vi "Batch Editor Dialog.vi"(5 "VI Refnum":refnum<vi>, 6 "Listbox":refnum<vi>, 7 "Reference":variant, 8 "Error in":errorcluster caption="Error in (no error)", 9 "Option":variant, 10 "Root":path, 11 "Entries":string[](array[string])) -> (0 "Error out":errorcluster)   [LabVIEW 2017, in "batchEditorDialog.lvlib"]
uses:
  batchEditorDialog.lvlib
  _Shared/CSM Shared.lvlib
panel:
  out "Listbox":i32(listbox)
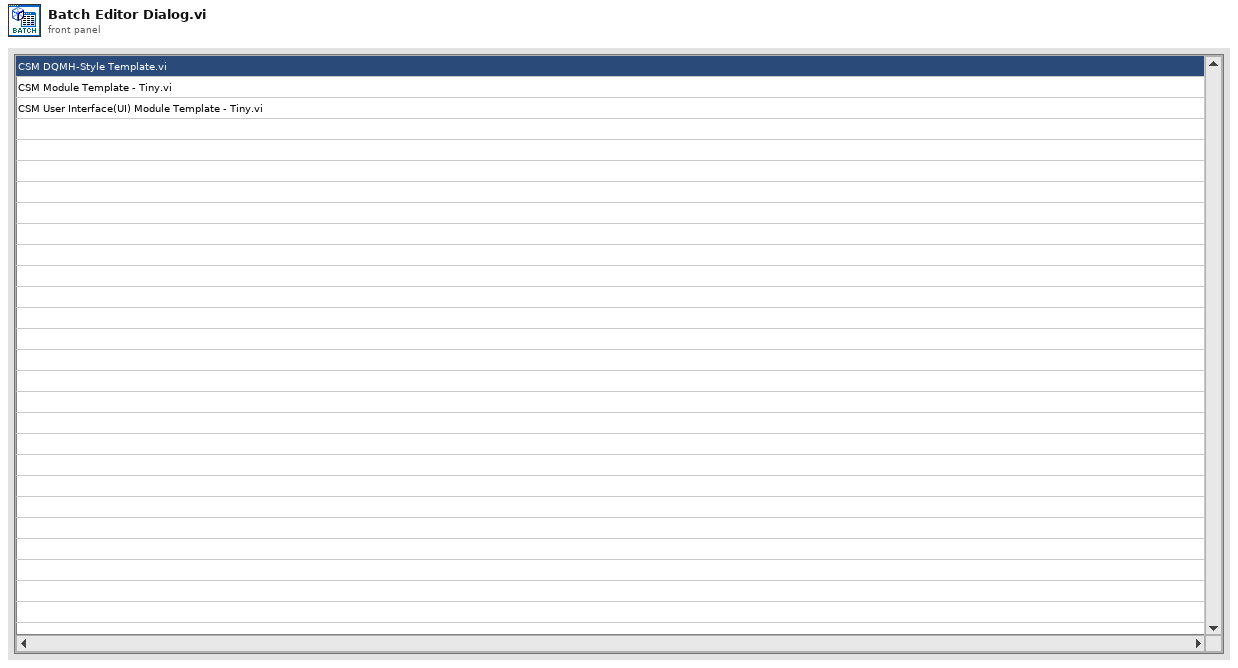
[diagram p1: front panel]
types:
  T1 = enum32{"Invalid", "Standard", "Closed", "Hidden", "Minimized", "Maximized"}
  T2 = enum32{"invalid app kind", "Development System", "Run Time System", "Student Edition", "Embedded LabVIEW", "Evaluation", "Custom"}
  T3 = cluster{"Core":cluster{"Current VI Reference":refnum<vi>, "Close Panel on Exit?":bool}, "Entries":string[], "Success":bool, "Listbox":refnum<vi>}
  T4 = cluster{"Current VI Reference":refnum<vi>, "Close Panel on Exit?":bool}
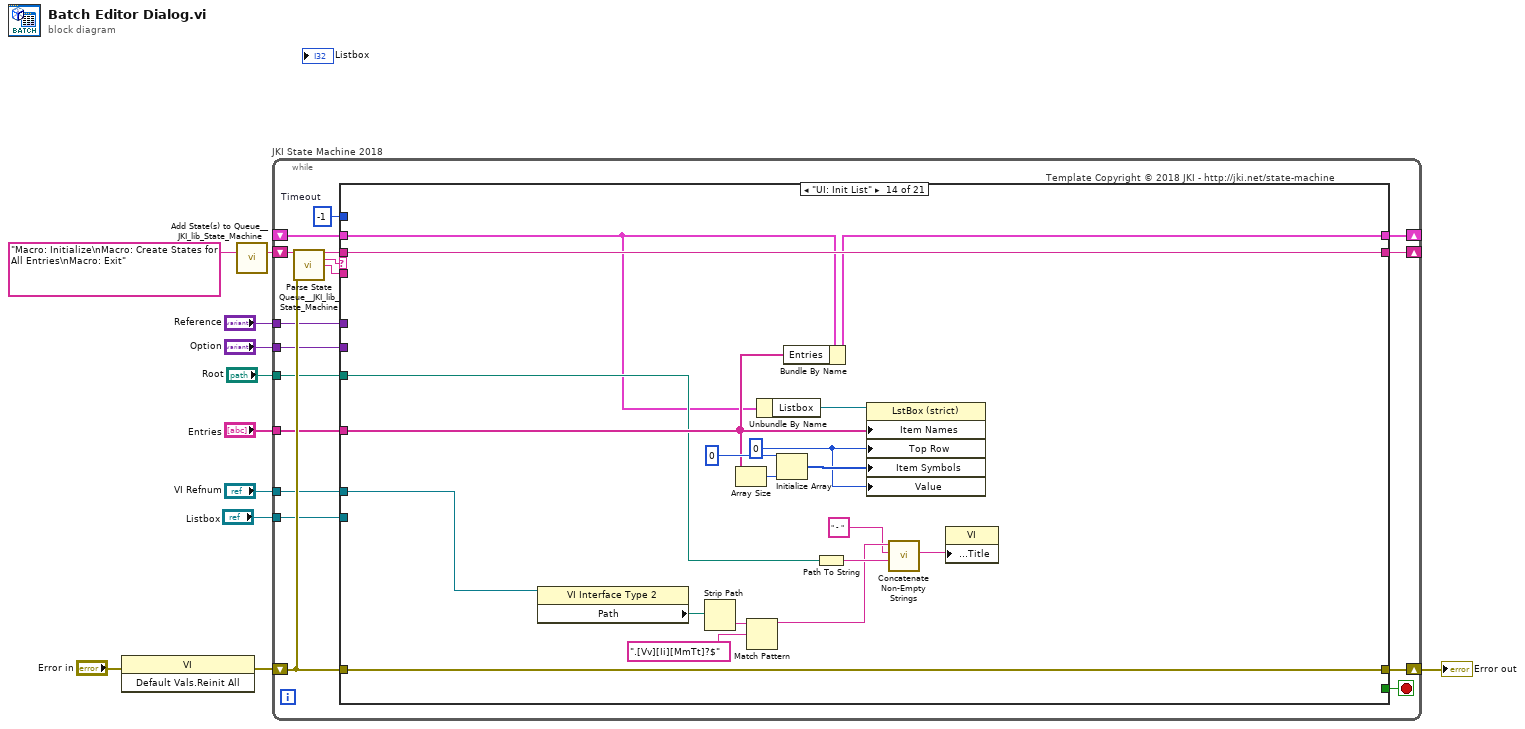
[diagram p0: block diagram]
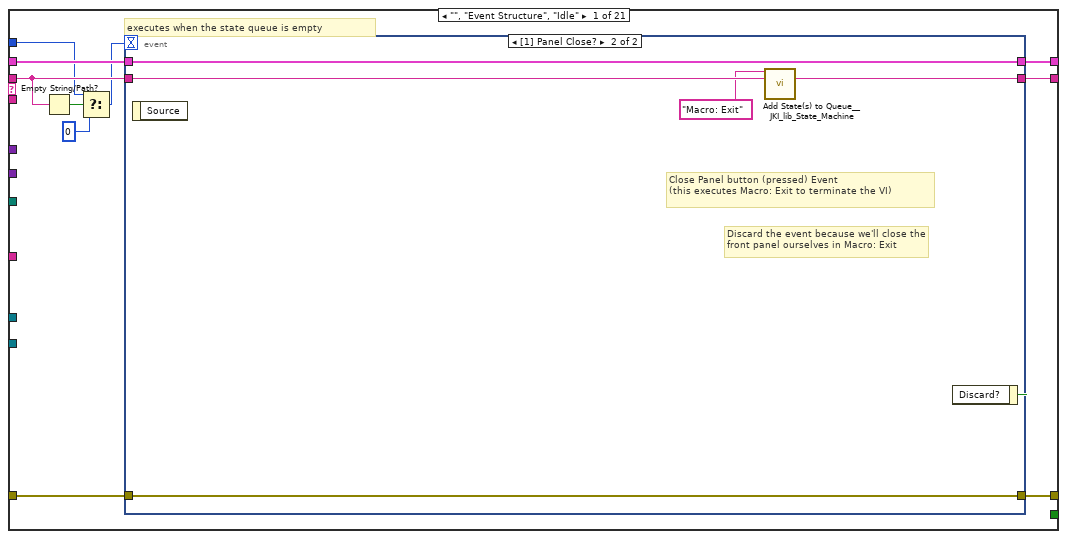
[diagram p2: hidden frame]
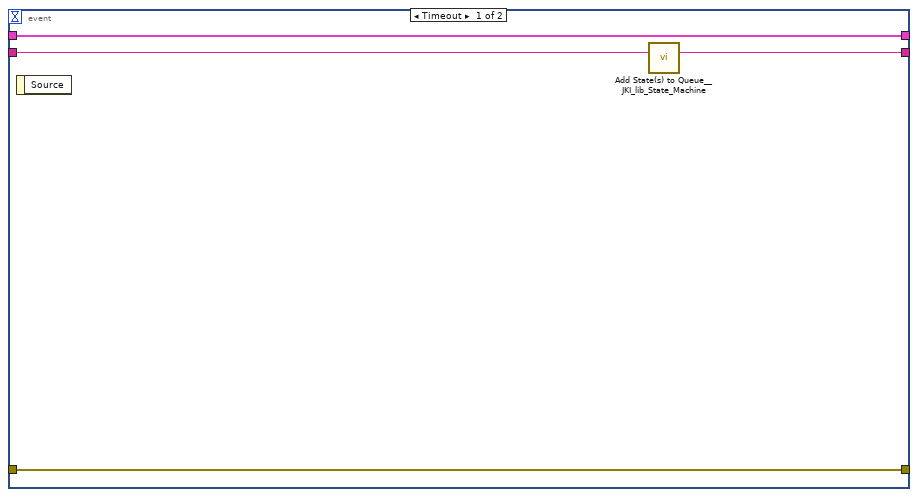
[diagram p3: hidden frame]
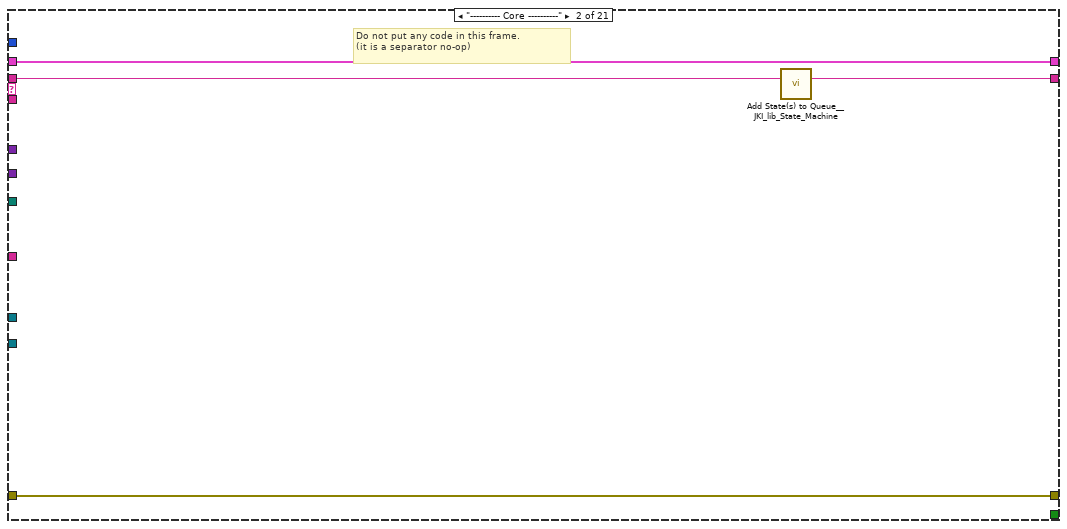
[diagram p4: hidden frame]
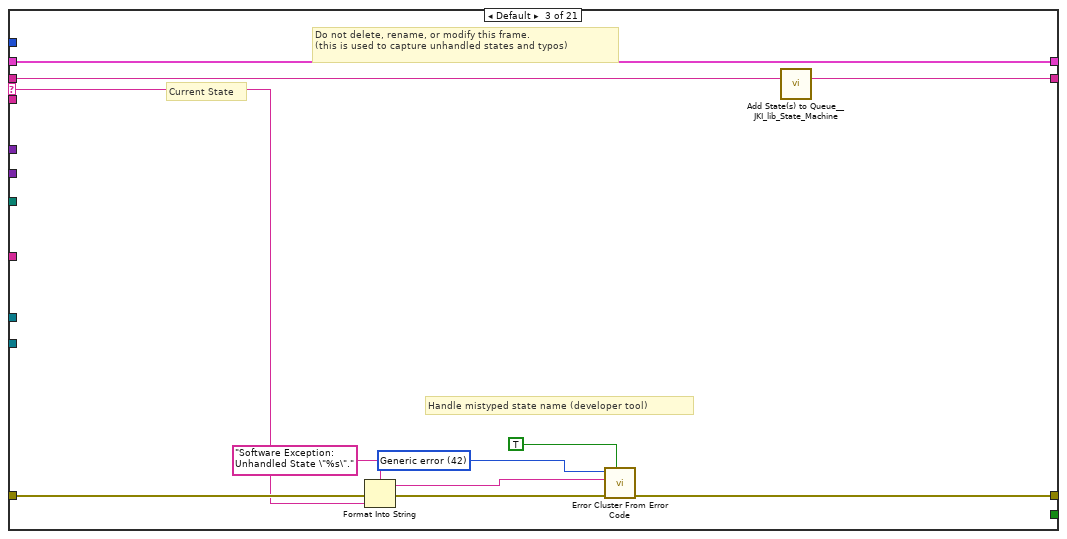
[diagram p5: hidden frame]
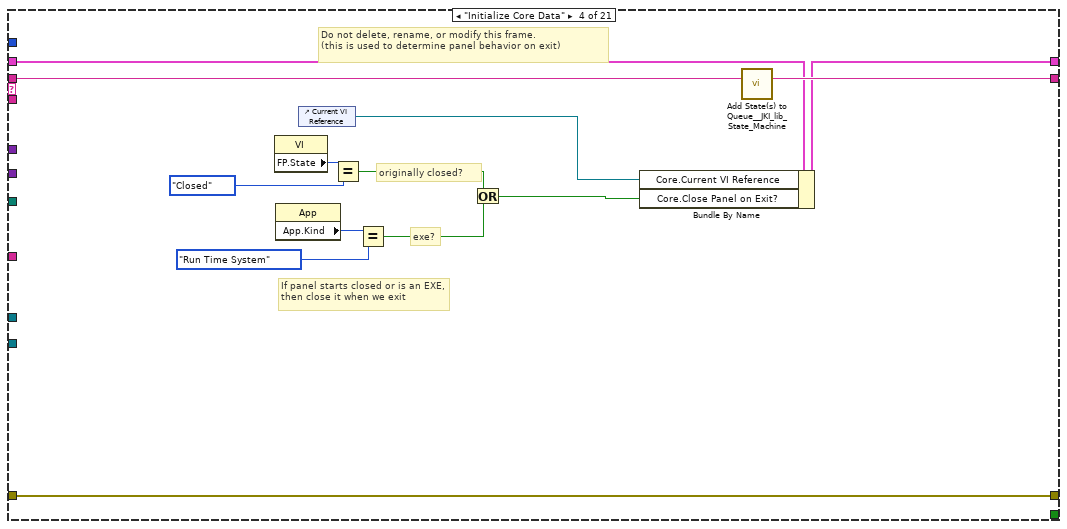
[diagram p6: hidden frame]
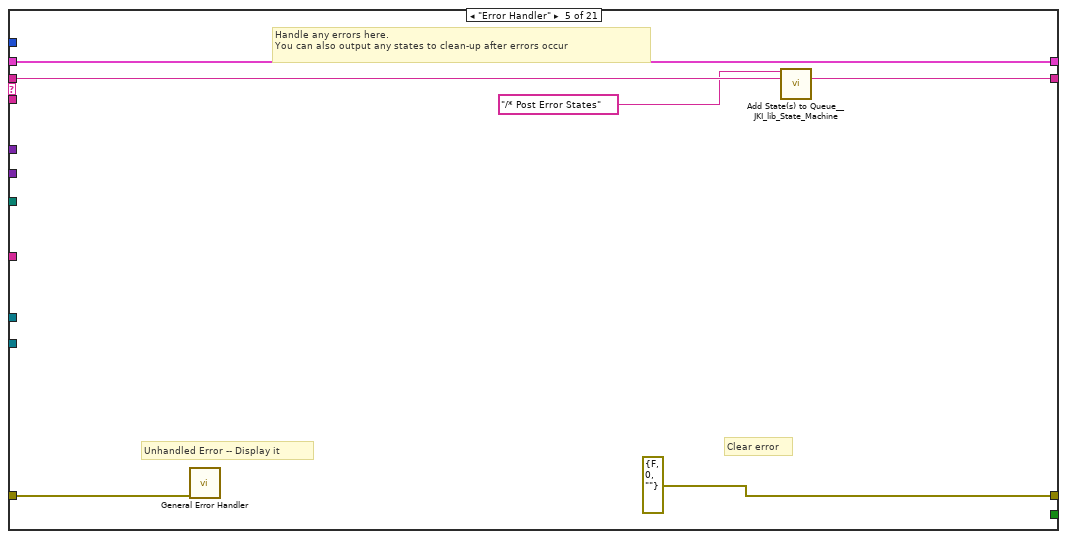
[diagram p7: hidden frame]
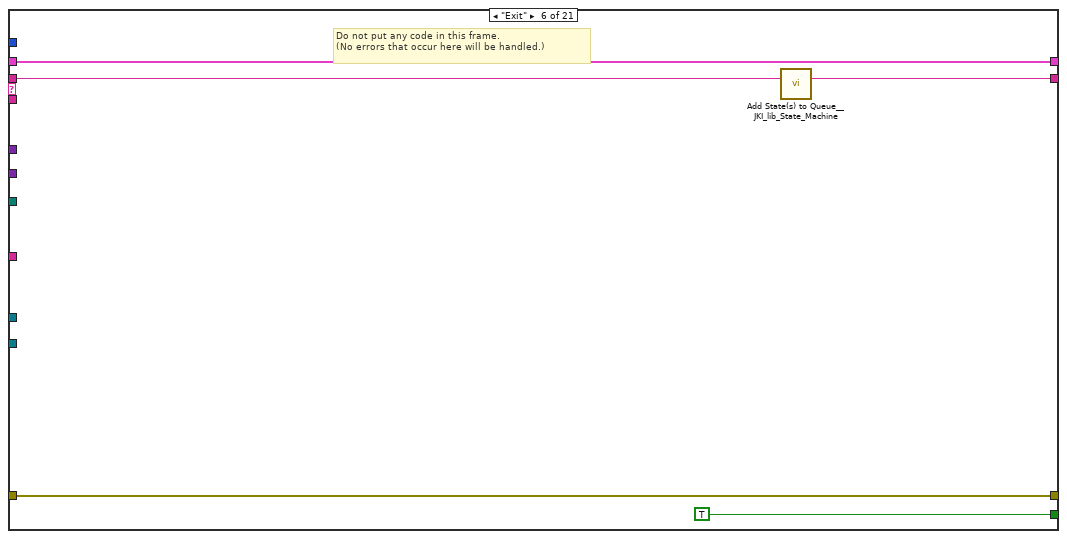
[diagram p8: hidden frame]
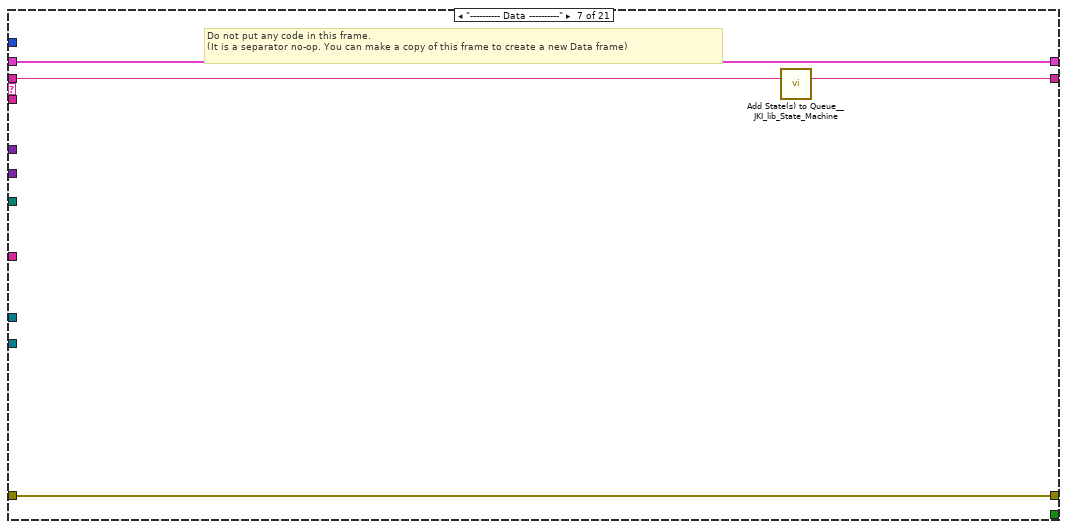
[diagram p9: hidden frame]
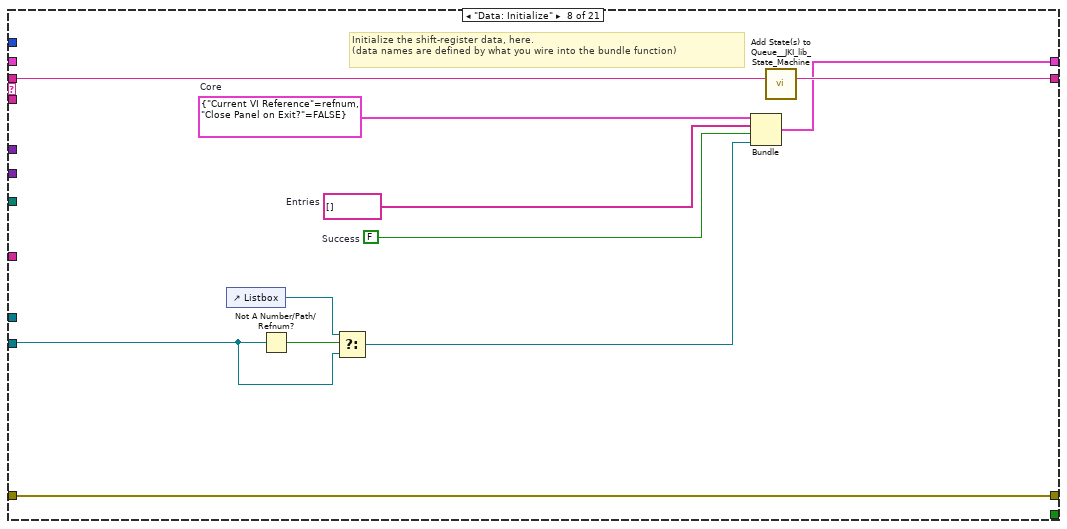
[diagram p10: hidden frame]
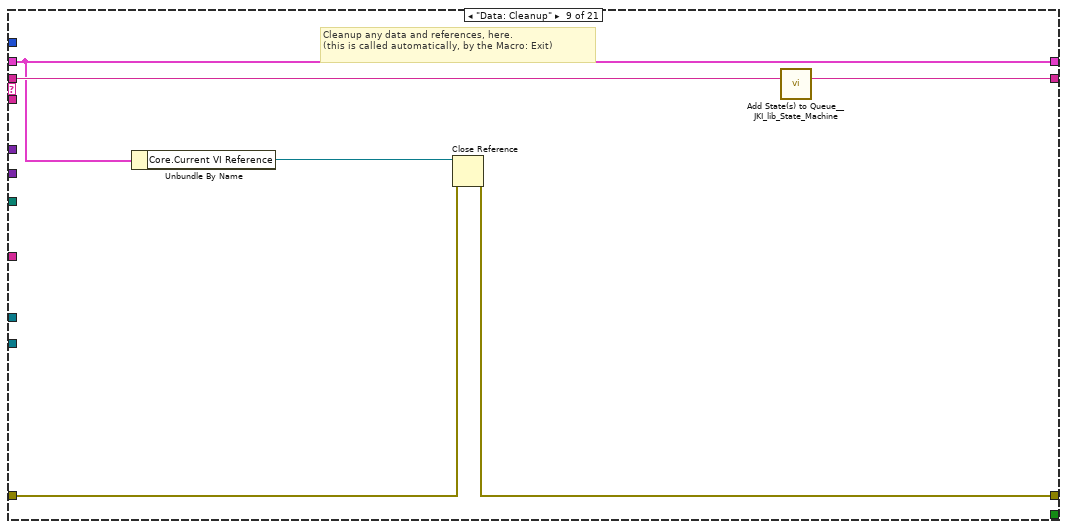
[diagram p11: hidden frame]
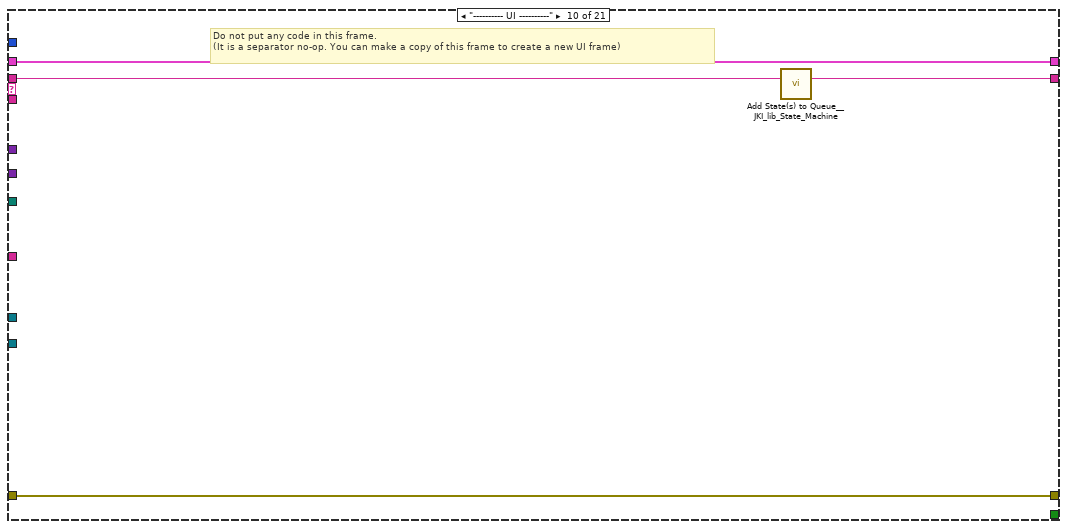
[diagram p12: hidden frame]
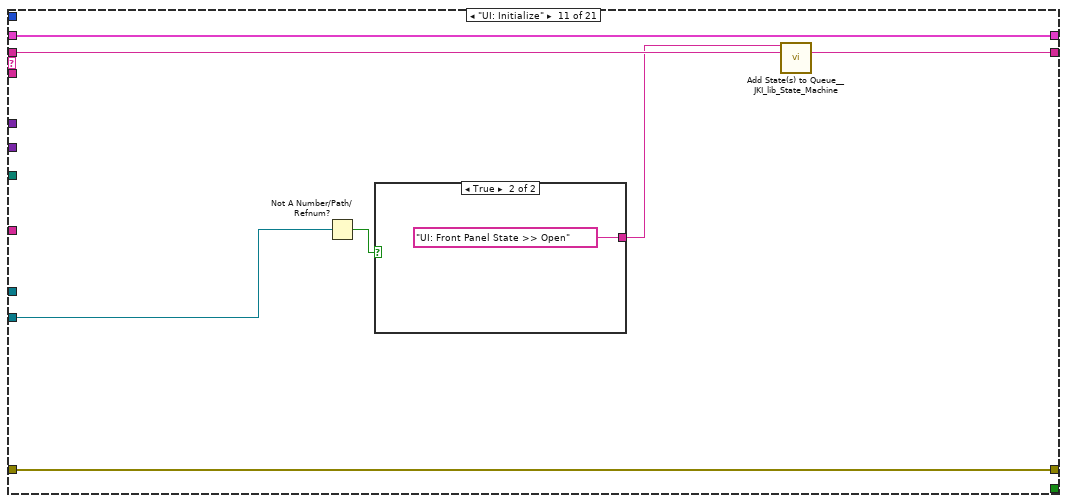
[diagram p13: hidden frame]
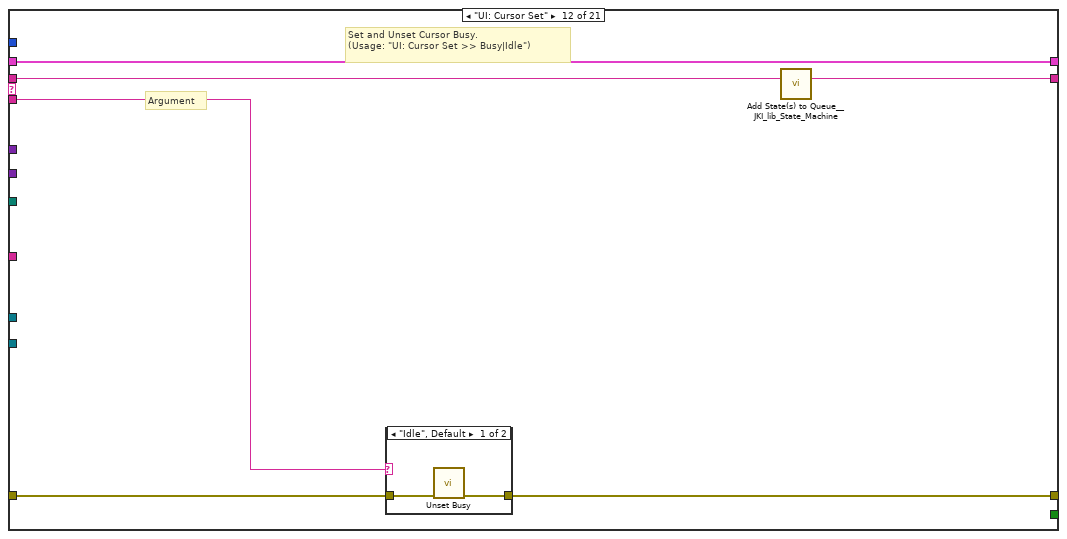
[diagram p15: hidden frame]
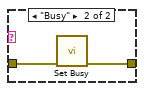
[diagram p16: hidden frame]
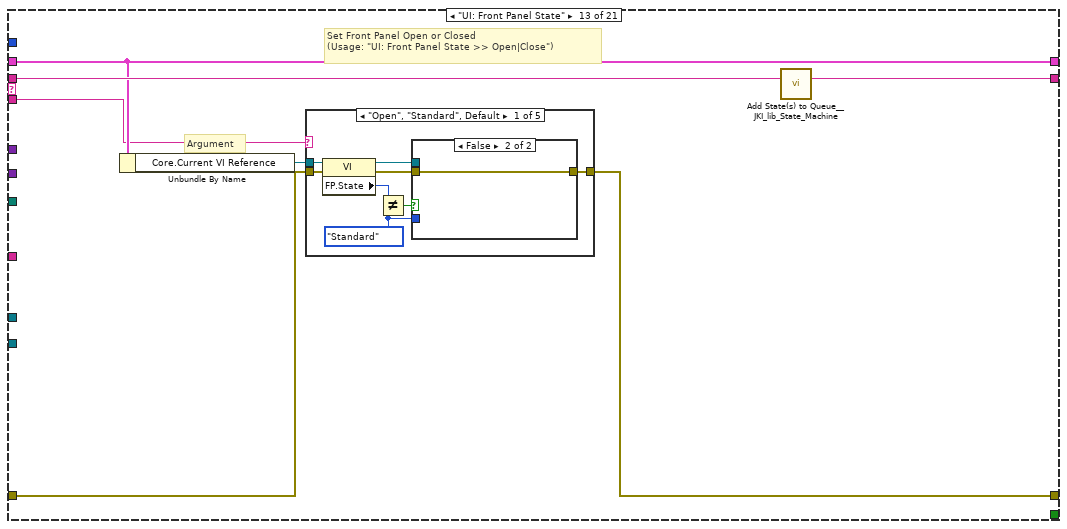
[diagram p17: hidden frame]
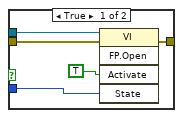
[diagram p18: hidden frame]
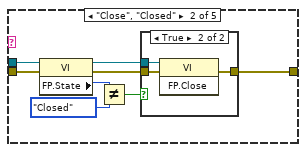
[diagram p19: hidden frame]
diagram:
  n1 = invoke class="VI" method="Default Vals.Reinit All"(error in="Error in") -> (error out=w9:errorcluster)  [unwired: 2 in, 2 out]
  n2 = call <vilib>:"Add State(s) to Queue__JKI_lib_State_Machine.vi"("State(s) in (\"\")"="Macro: Initialize\nMacro: Create States for All Entries\nMacro: Exit") -> ("States Out"=w11:string)  [unwired: 14 in]
  n3 = while "JKI State Machine 2018" {
    shift-right: [w21] -> _
    shift-left: _ -> [w20]
    shift-right: [w24] -> w7
    shift-left: w9 -> [w18]
    shift-right: [w23] -> _
    shift-left: w11 -> [w25]
    tunnel: "Reference" -> [w17]
    tunnel: "Option" -> [w16]
    tunnel: "Entries" -> [w15]
    tunnel: "VI Refnum" -> [w14]
    tunnel: "Root" -> [w13]
    tunnel: "Listbox" -> [w12]
    stop <- w22 stop-if-true
    w19 = -1  # Timeout
    # "Template Copyright © 2018 JKI - http://jki.net/state-machine"
    n4 = call <vilib>:"Parse State Queue__JKI_lib_State_Machine.vi"("State Queue"=w25, "Error In (no error)"=w18) -> ("Remaining States"=w27:string, "Current State"=w28:string, "Arguments"=w26:string)  [unwired: 11 in]
    n5 = case shown="\"UI: Init List\"" w28 {
      selector: w28 -> [_ _ w53 _ _ _ _ _ _ _ _ _ _ _ _ _ _ _ _ _ _]
      tunnel: w27 -> [w33 w52 w57 w76 w82 w87 w91 w102 w108 w112 w119 w126 w137 w220 w225 w247 w252 w262 w266 w274 w292]
      tunnel: w26 -> [_ _ _ _ _ _ _ _ _ _ _ w121 w131 _ _ _ _ _ _ _ w286]
      tunnel: w20 -> [w37 w49 w55 w69 w79 w85 w88 _ w103 w109 w116 w124 w133 w212 w223 w244 w249 w259 w263 w270 w290]
      tunnel: [w36 w50 w59 w73 errorcluster {"status"=FALSE, "code"=0, "source"=""} ("error out") w84 w89 w99 w104 w110 w117 w122 w134 w221 w243 w245 w250 w260 w264 w272 _] -> w24
      tunnel: w18 -> [w35 w50 w58 w73 w78 w84 w89 w99 w105 w110 w117 w123 w135 w221 w243 w245 w250 w260 w264 w272 _]
      tunnel: [w38 w51 w56 w75 w81 w86 w90 w101 w107 w111 w118 w125 w136 w220 w226 w246 w251 w261 w265 w273 w293] -> w23
      tunnel: [_ _ _ _ _ TRUE _ _ _ _ _ _ _ _ _ _ _ _ _ _ _] -> w22
      tunnel: [w34 w49 w55 w74 w79 w85 w88 w100 w103 w109 w116 w124 w133 w215 w232 w244 w249 w259 w263 w270 w295] -> w21
      tunnel: w19 -> [w32 _ _ _ _ _ _ _ _ _ _ _ _ _ _ _ _ _ _ _ _]
      tunnel: w17 -> [_ _ _ _ _ _ _ _ _ _ _ _ _ _ _ _ _ _ _ _ w285]
      tunnel: w16 -> [_ _ _ _ _ _ _ _ _ _ _ _ _ _ _ _ _ _ _ _ w284]
      tunnel: w15 -> [_ _ _ _ _ _ _ _ _ _ _ _ _ w214 _ _ _ _ _ _ _]
      tunnel: w14 -> [_ _ _ _ _ _ _ _ _ _ _ _ _ w210 _ _ _ _ _ _ w283]
      tunnel: w13 -> [_ _ _ _ _ _ _ _ _ _ _ _ _ w213 _ _ _ _ _ _ w281]
      tunnel: w12 -> [_ _ _ _ _ _ _ w93 _ _ w114 _ _ _ _ _ _ _ _ _ _]
      frame "", "Event Structure", "Idle" {
        # "executes when the state queue is empty"
        n6 = Empty String/Path?(string/path=w33) -> (empty?=w30:bool)
        n7 = Select(t=w32, s=w30, f=0) -> (s? t:f=w31:i32)
        n8 = event shown="[1] Panel Close?" {
          selector: _ -> [_ _]
          dyn-events: _ -> [_ _]
          timeout: w31 -> [_ _]
          tunnel: w33 -> [w42 w48]
          tunnel: [w41 w47] -> w38
          tunnel: w37 -> [w39 w45]
          tunnel: [w40 w46] -> w36
          tunnel: w35 -> [w40 w46]
          tunnel: [w39 w45] -> w34
          event Timeout {
            n9 = event-data() -> ()  [unwired: 1 in, 1 out]
            n10 = call <vilib>:"Add State(s) to Queue__JKI_lib_State_Machine.vi"("State(s) in (\"\")"=w42) -> ("States Out"=w41:string)  [unwired: 14 in]
          }
          event Panel Close? {
            # "Discard the event because we'll close the front panel ourselves in Macro: Exit"
            # "Close Panel button (pressed) Event\n(this executes Macro: Exit to terminate the VI)"
            n11 = event-data() -> ()  [unwired: 1 in, 1 out]
            n12 = call <vilib>:"Add State(s) to Queue__JKI_lib_State_Machine.vi"("State(s) in Front (\"\")"="Macro: Exit", "State(s) in (\"\")"=w48) -> ("States Out"=w47:string)  [unwired: 13 in]
            n13 = event-data("Discard?"=TRUE) -> ()  [unwired: 1 in, 1 out]
          }
        }
      }
      frame "---------- Core ----------" {
        # "Do not put any code in this frame.\n(it is a separator no-op)"
        n14 = call <vilib>:"Add State(s) to Queue__JKI_lib_State_Machine.vi"("State(s) in (\"\")"=w52) -> ("States Out"=w51:string)  [unwired: 14 in]
      }
      frame Default {
        w62 = 42 items=["No error", "Argument error", "Memory is full", "Out of zone", "End of file", "File already open", "Generic file I/O error", "File not found", "File permission error", "Disk is full", "Duplicate path", "Too many files open", "System feature not enabled", "Resource file not found", "Cannot add resource", "Resource not found", "Image not found", "Image memory error", "Pen does not exist", "Config type invalid", "Config token not found", "Config parse error", "Config memory error", "Bad external code format", "Bad external code offset", "External code not present", "Null window", "Destroy window error", "Null menu", "Print aborted", "Bad print record", "Print driver error", "Windows error during printing", "Memory error during printing", "Print dialog error", "Generic print error", "Invalid device refnum", "Device not found", "Device parameter error", "Device unit error", "Cannot open device", "Device call aborted", "Generic error", "Cancelled by user", "Object ID too low", "Object ID too high", "Object not in heap", "Unknown heap", "Unknown object (invalid DefProc)", "Unknown object (DefProc not in table)", "Message out of range", "Invalid (null) method", "Unknown message", "Manager call not supported", "Bad address", "Network operation in progress", "Network operation timed out", "Connection is busy", "Network attribute not supported", "Network error", "Address in use", "System out of memory", "Connection aborted", "Connection refused", "Not connected", "Already connected", "Connection closed", "Initialization error (interapplication manager)", "Bad occurrence", "Wait on unbound occurrence handler", "Occurrence queue overflow", "Datalog type conflict", "Unused", "Unrecognized type (interapplication manager)", "Memory corrupt", "Failed to make temporary DLL", "Old CIN version", "Drag socket not found", "Failed to load drop-object", "Failed to register OLE object", "Failed to release OLE object", "Format specifier type mismatch", "Unknown format specifier", "Too few format specifiers", "Too many format specifiers", "Scan failed", "Newer CIN version", "Error converting to variant", "Runtime menu error", "Password tampered", "Variant attribute not found", "Incompatible variant data type", "Event data is not available", "Event Store is not present", "Occurrence is not found", "Event Queue is not created", "Event info is not available", "Refnum passed is NULL", "Error retrieving Class GUID", "Error retrieving CoClass GUID", "Error retrieving TypeLib GUID.", "Bad built application magic bytes.", "Specific driver is different from the specific driver associated with the Logical Name.", "There is no session opened to the class driver.", "Max Error", "MAX - Error with config objects", "MAX - Error loading configuration", "MAX - Group not supported"]
        # "Current State"
        # "Do not delete, rename, or modify this frame.\n(this is used to capture unhandled states and typos)"
        # "Handle mistyped state name (developer tool)"
        n15 = Format Into String(format string="Software Exception: Unhandled State \"%s\"." ("message"), error in=w58, w53) -> (resulting string=w61:string, error out=w60:errorcluster)  [unwired: 1 in]
        n16 = call <vilib>:"Error Cluster From Error Code.vi"("show call chain? (False)"=TRUE, "error in (no error)"=w60, "error message (\"\")"=w61, "error code (0)"=w62) -> ("error out"=w59:errorcluster)  [unwired: 5 in]
        n17 = call <vilib>:"Add State(s) to Queue__JKI_lib_State_Machine.vi"("State(s) in (\"\")"=w57) -> ("States Out"=w56:string)  [unwired: 14 in]
      }
      frame "Initialize Core Data" {
        # "Do not delete, rename, or modify this frame.\n(this is used to determine panel behavior on exit)"
        # "originally closed?"
        # "exe?"
        # "If panel starts closed or is an EXE, then close it when we exit"
        n18 = property class="VI"() -> ("FP.State"=w66:T1)  [unwired: 2 in, 2 out]
        n19 = property class="App"() -> ("App.Kind"=w72:T2)  [unwired: 2 in, 2 out]
        n20 = control-ref of="Current VI Reference"() -> (w67:refnum<vi>)
        n21 = Equal?(x=w66, y=T1."Closed" ("Front Panel Window:State")) -> (x = y?=w64:bool)
        n22 = Equal?(x=w72, y=T2."Run Time System" ("Application:Kind")) -> (x = y?=w70:bool)
        n23 = Or(x=w64, y=w70) -> (x .or. y?=w68:bool)
        n24 = Bundle By Name(cluster=w69, "Core.Current VI Reference"=w67, "Core.Close Panel on Exit?"=w68) -> (w74:T3)
        n25 = call <vilib>:"Add State(s) to Queue__JKI_lib_State_Machine.vi"("State(s) in (\"\")"=w76) -> ("States Out"=w75:string)  [unwired: 14 in]
      }
      frame "Error Handler" {
        # "Unhandled Error -- Display it"
        # "Handle any errors here.\nYou can also output any states to clean-up after errors occur"
        # "Clear error"
        n26 = call <vilib>:"General Error Handler.vi"("error in (no error)"=w78) -> ()  [unwired: 10 in, 5 out]
        n27 = call <vilib>:"Add State(s) to Queue__JKI_lib_State_Machine.vi"("State(s) in Front (\"\")"="/* Post Error States", "State(s) in (\"\")"=w82) -> ("States Out"=w81:string)  [unwired: 13 in]
      }
      frame "Exit" {
        # "Do not put any code in this frame.\n(No errors that occur here will be handled.)"
        n28 = call <vilib>:"Add State(s) to Queue__JKI_lib_State_Machine.vi"("State(s) in (\"\")"=w87) -> ("States Out"=w86:string)  [unwired: 14 in]
      }
      frame "---------- Data ----------" {
        # "Do not put any code in this frame.\n(It is a separator no-op. You can make a copy of this frame to create a new Data frame)"
        n29 = call <vilib>:"Add State(s) to Queue__JKI_lib_State_Machine.vi"("State(s) in (\"\")"=w91) -> ("States Out"=w90:string)  [unwired: 14 in]
      }
      frame "Data: Initialize" {
        w96 = FALSE  # Success
        w97 = string[] []  # Entries
        w98 = T4 {"Current VI Reference"=refnum, "Close Panel on Exit?"=FALSE}  # Core
        # "Initialize the shift-register data, here.\n(data names are defined by what you wire into the bundle function)"
        n30 = control-ref of="Listbox"() -> (w94:refnum<vi>)
        n31 = Not A Number/Path/Refnum?(number/path/refnum=w93) -> (NaN/Path/Refnum?=w95:bool)
        n32 = Select(t=w94, s=w95, f=w93) -> (s? t:f=w92:refnum<vi>)
        n33 = Bundle("Core"=w98, "Entries"=w97, "Success"=w96, "Listbox"=w92) -> (w100:T3)  [unwired: 1 in]
        n34 = call <vilib>:"Add State(s) to Queue__JKI_lib_State_Machine.vi"("State(s) in (\"\")"=w102) -> ("States Out"=w101:string)  [unwired: 14 in]
      }
      frame "Data: Cleanup" {
        # "Cleanup any data and references, here.\n(this is called automatically, by the Macro: Exit)"
        n35 = Unbundle By Name(w103) -> ("Core.Current VI Reference"=w106:refnum<vi>)
        n36 = Close Reference(reference=w106, error in (no error)=w105) -> (error out=w104:errorcluster)
        n37 = call <vilib>:"Add State(s) to Queue__JKI_lib_State_Machine.vi"("State(s) in (\"\")"=w108) -> ("States Out"=w107:string)  [unwired: 14 in]
      }
      frame "---------- UI ----------" {
        # "Do not put any code in this frame.\n(It is a separator no-op. You can make a copy of this frame to create a new UI frame)"
        n38 = call <vilib>:"Add State(s) to Queue__JKI_lib_State_Machine.vi"("State(s) in (\"\")"=w112) -> ("States Out"=w111:string)  [unwired: 14 in]
      }
      frame "UI: Initialize" {
        n39 = Not A Number/Path/Refnum?(number/path/refnum=w114) -> (NaN/Path/Refnum?=w113:bool)
        n40 = case shown="True" w113 {
          tunnel: [_ "UI: Front Panel State >> Open" ("State(s) in Front (\"\")")] -> w115
          frame False {
          }
          frame True {
          }
        }
        n41 = call <vilib>:"Add State(s) to Queue__JKI_lib_State_Machine.vi"("State(s) in Front (\"\")"=w115, "State(s) in (\"\")"=w119) -> ("States Out"=w118:string)  [unwired: 13 in]
      }
      frame "UI: Cursor Set" {
        # "Argument"
        # "Set and Unset Cursor Busy.\n(Usage: \"UI: Cursor Set >> Busy|Idle\")"
        n42 = case shown="\"Idle\", Default" w121 {
          tunnel: w123 -> [w128 w130]
          tunnel: [w127 w129] -> w122
          frame "Idle", Default {
            n43 = call <vilib>:"Unset Busy.vi"("error in (no error)"=w128) -> ("error out"=w127:errorcluster)  [unwired: 10 in]
          }
          frame "Busy" {
            n44 = call <vilib>:"Set Busy.vi"("error in (no error)"=w130) -> ("error out"=w129:errorcluster)  [unwired: 9 in, 1 out]
          }
        }
        n45 = call <vilib>:"Add State(s) to Queue__JKI_lib_State_Machine.vi"("State(s) in (\"\")"=w126) -> ("States Out"=w125:string)  [unwired: 14 in]
      }
      frame "UI: Front Panel State" {
        # "Argument"
        # "Set Front Panel Open or Closed\n(Usage: \"UI: Front Panel State >> Open|Close\")"
        n46 = Unbundle By Name(w133) -> ("Core.Current VI Reference"=w132:refnum<vi>)
        n47 = case shown="\"Open\", \"Standard\", Default" w131 {
          tunnel: w135 -> [w143 w158 w169 w182 w195]
          tunnel: [w145 w159 w171 w184 w197] -> w134
          tunnel: w132 -> [w144 w156 w170 w183 w196]
          frame "Open", "Standard", Default {
            w138 = T1."Standard" ("State")
            n48 = property class="VI"(reference=w144, error in=w143) -> (reference out=w141:refnum<vi>, error out=w142:errorcluster, "FP.State"=w140:T1)
            n49 = Not Equal?(x=w140, y=w138) -> (x != y?=w139:bool)
            n50 = case shown="False" w139 {
              tunnel: [w149 w151] -> w145
              tunnel: w142 -> [w148 w151]
              tunnel: w141 -> [w147 _]
              tunnel: w138 -> [w146 _]
              frame True {
                n51 = invoke class="VI" method="FP.Open"(reference=w147, error in=w148, "Activate"=TRUE, "State"=w146) -> (error out=w149:errorcluster)  [unwired: 1 in, 4 out]
              }
              frame False {
              }
            }
          }
          frame "Close", "Closed" {
            n52 = property class="VI"(reference=w156, error in=w158) -> (reference out=w155:refnum<vi>, error out=w157:errorcluster, "FP.State"=w153:T1)
            n53 = Not Equal?(x=w153, y=T1."Closed" ("Front Panel Window:State")) -> (x != y?=w152:bool)
            n54 = case shown="True" w152 {
              tunnel: [w160 w163] -> w159
              tunnel: w157 -> [w160 w162]
              tunnel: w155 -> [_ w161]
              frame False {
              }
              frame True {
                n55 = invoke class="VI" method="FP.Close"(reference=w161, error in=w162) -> (error out=w163:errorcluster)  [unwired: 1 in, 2 out]
              }
            }
          }
          frame "Hidden", "Hide" {
            w164 = T1."Hidden" ("State")
            n56 = property class="VI"(reference=w170, error in=w169) -> (reference out=w167:refnum<vi>, error out=w168:errorcluster, "FP.State"=w166:T1)
            n57 = Not Equal?(x=w166, y=w164) -> (x != y?=w165:bool)
            n58 = case shown="True" w165 {
              tunnel: [w175 w176] -> w171
              tunnel: w168 -> [w174 w176]
              tunnel: w167 -> [w173 _]
              tunnel: w164 -> [w172 _]
              frame True {
                n59 = invoke class="VI" method="FP.Open"(reference=w173, error in=w174, "State"=w172) -> (error out=w175:errorcluster)  [unwired: 2 in, 4 out]
              }
              frame False {
              }
            }
          }
          frame "Minimize", "Minimized" {
            w177 = T1."Minimized" ("State")
            n60 = property class="VI"(reference=w183, error in=w182) -> (reference out=w180:refnum<vi>, error out=w181:errorcluster, "FP.State"=w179:T1)
            n61 = Not Equal?(x=w179, y=w177) -> (x != y?=w178:bool)
            n62 = case shown="True" w178 {
              tunnel: [w188 w189] -> w184
              tunnel: w181 -> [w187 w189]
              tunnel: w180 -> [w186 _]
              tunnel: w177 -> [w185 _]
              frame True {
                n63 = invoke class="VI" method="FP.Open"(reference=w186, error in=w187, "State"=w185) -> (error out=w188:errorcluster)  [unwired: 2 in, 4 out]
              }
              frame False {
              }
            }
          }
          frame "Maximize", "Maximized" {
            w190 = T1."Maximized" ("State")
            n64 = property class="VI"(reference=w196, error in=w195) -> (reference out=w193:refnum<vi>, error out=w194:errorcluster, "FP.State"=w192:T1)
            n65 = Not Equal?(x=w192, y=w190) -> (x != y?=w191:bool)
            n66 = case shown="True" w191 {
              tunnel: [w201 w202] -> w197
              tunnel: w194 -> [w200 w202]
              tunnel: w193 -> [w199 _]
              tunnel: w190 -> [w198 _]
              frame True {
                n67 = invoke class="VI" method="FP.Open"(reference=w199, error in=w200, "State"=w198) -> (error out=w201:errorcluster)  [unwired: 2 in, 4 out]
              }
              frame False {
              }
            }
          }
        }
        n68 = call <vilib>:"Add State(s) to Queue__JKI_lib_State_Machine.vi"("State(s) in (\"\")"=w137) -> ("States Out"=w136:string)  [unwired: 14 in]
      }
      frame "UI: Init List" {
        w216 = 0 ("Top Row")
        n69 = property class="VI Interface Type 2"(reference=w210) -> ("Path"=w209:path)  [unwired: 1 in, 2 out]
        n70 = Strip Path(path=w209) -> (name=w208:string)  [unwired: 1 out]
        n71 = Array Size(array=w214) -> (size(s)=w219:i32)
        n72 = Match Pattern(string=w208, regular expression=".[Vv][Ii][MmTt]?$") -> (before substring=w204:string)  [unwired: 1 in, 3 out]
        n73 = Unbundle By Name(w212) -> ("Listbox"=w211:refnum<vi>)
        n74 = Initialize Array(0 ("Top Row"), w219) -> (w217:i32[])
        n75 = Bundle By Name(cluster=w212, "Entries"=w214) -> (w215:T3)
        n76 = Path To String(path=w213) -> (string=w205:string)
        n77 = property on="Property Node" class="LstBox (strict)"(reference=w211, "Item Names"=w214, "Top Row"=w216, "Item Symbols"=w217, "Value"=w216) -> ()  [unwired: 1 in, 2 out]
        n78 = call "Concatenate Non-Empty Strings.vi"("String2"=w205, "Seperator(Carriage Return)"=" - " ("string"), "String1"=w204) -> ("Result String"=w206:string)  [unwired: 5 in]
        n79 = property class="VI"("Front Panel.Title"=w206) -> ()  [unwired: 2 in, 2 out]
      }
      frame "UI: Post Action" {
        n80 = Unbundle By Name(w223) -> ("Listbox"=w222:refnum<vi>)
        n81 = Unbundle By Name(w223) -> ("Success"=w230:bool)
        n82 = property on="Property Node" class="LstBox (strict)"(reference=w222) -> (reference out=w234:refnum<vi>, error out=w233:errorcluster, "Value"=w235:i32, "Item Symbols"=w242:i32[])  [unwired: 1 in]
        n83 = Select(t=1 ("new element/subarray"), s=w230, f=2 ("new element/subarray")) -> (s? t:f=w227:i32)
        n84 = Replace Array Subset(array=w242, new element=w227, index=w235) -> (w241:i32[])
        n85 = Subtract(x=w235, y=5) -> (x-y=w238:i32)
        n86 = Increment(x=w235) -> (x+1=w240:i32)
        n87 = Max & Min(x=w238, y=0) -> (max(x,y)=w236:i32)  [unwired: 1 out]
        n88 = property on="Property Node" class="LstBox (strict)"(reference=w234, error in=w233, "Top Row"=w236, "Item Symbols"=w241, "Value"=w240) -> ()  [unwired: 2 out]
        n89 = Bundle By Name(cluster=w223, "Success"=TRUE ("Last Action Success")) -> (w232:T3)
        n90 = call <vilib>:"Add State(s) to Queue__JKI_lib_State_Machine.vi"("State(s) in Front (\"\")"="Idle" ("State(s) in Front (\"\")"), "State(s) in (\"\")"=w225) -> ("States Out"=w226:string)  [unwired: 13 in]
      }
      frame "---------- Macro ----------" {
        # "Do not put any code in this frame.\n(It is a separator no-op. You can make a copy of this frame to create a new Macro frame)"
        n91 = call <vilib>:"Add State(s) to Queue__JKI_lib_State_Machine.vi"("State(s) in (\"\")"=w247) -> ("States Out"=w246:string)  [unwired: 14 in]
      }
      frame "Macro: Initialize" {
        # "Initialization Macro\n(This is called once, when the VI starts)"
        n92 = call <vilib>:"Add State(s) to Queue__JKI_lib_State_Machine.vi"("State(s) in Front (\"\")"="Data: Initialize\nInitialize Core Data\nUI: Initialize\n//UI: Front Panel State >> Open\nUI: Init List", "State(s) in (\"\")"=w252) -> ("States Out"=w251:string)  [unwired: 13 in]
      }
      frame "Macro: Exit" {
        n93 = Unbundle By Name(w259) -> ("Core.Close Panel on Exit?"=w258:bool)
        n94 = Select(t="UI: Front Panel State >> Close", s=w258, f="") -> (s? t:f=w255:string)
        n95 = call <vilib>:"Add State(s) to Queue__JKI_lib_State_Machine.vi"("State(s) in (\"\")"=w255, "State(s) at Back (\"\")"="Data: Cleanup\nExit") -> ("States Out"=w253:string)  [unwired: 13 in]
        n96 = call <vilib>:"Add State(s) to Queue__JKI_lib_State_Machine.vi"("State(s) in Front (\"\")"=w253, "State(s) in (\"\")"=w262) -> ("States Out"=w261:string)  [unwired: 13 in]
      }
      frame "---------- Action ----------" {
        # "Template Separator\n(You can make a copy of, or modify, this frame)"
        n97 = call <vilib>:"Add State(s) to Queue__JKI_lib_State_Machine.vi"("State(s) in (\"\")"=w266) -> ("States Out"=w265:string)  [unwired: 14 in]
      }
      frame "Macro: Create States for All Entries" {
        n98 = Unbundle By Name(w270) -> ("Entries"=w269:string[])
        n99 = for {
          tunnel: w269 -> [w279] mode=indexing
          tunnel: "Action: Process" ("State") -> [w278]
          shift-right: [w277] -> w267
          shift-left: "" ("State") -> [w276]
          n100 = call <vilib>:"Build State String with Arguments__JKI_lib_State_Machine.vi"("Arguments (\"\")"=w279, "State"=w278) -> ("State with Arguments"=w275:string)  [unwired: 4 in]
          n101 = call <vilib>:"Add State(s) to Queue__JKI_lib_State_Machine.vi"("State(s) in (\"\")"=w276, "State(s) at Back (\"\")"=w275) -> ("States Out"=w277:string)  [unwired: 13 in]
        }
        n102 = call <vilib>:"Add State(s) to Queue__JKI_lib_State_Machine.vi"("State(s) in Front (\"\")"=w267, "State(s) in (\"\")"=w274) -> ("States Out"=w273:string)  [unwired: 13 in]
      }
      frame "Action: Process" {
        n103 = Empty String/Path?(string/path=w281) -> (empty?=w280:bool)
        n104 = case shown="False" w280 {
          tunnel: w286 -> [w299 w300]
          tunnel: [w297 w300] -> w282
          tunnel: w281 -> [w296 _]
          frame False {
            n105 = Build Path(base path=w296, name or relative path=w299) -> (appended path=w298:path)
            n106 = Path To String(path=w298) -> (string=w297:string)
          }
          frame True {
          }
        }
        n107 = call-by-ref "?"(reference=w283, "Reference"=w285, "Option"=w284, "Entry"=w282) -> (error out=w289:errorcluster, "Error out"=w287:errorcluster)  [unwired: 9 in, 1 out]
        n108 = Merge Errors(w289, w287) -> (w288:errorcluster)
        n109 = call <vilib>:"Add State(s) to Queue__JKI_lib_State_Machine.vi"("State(s) in Front (\"\")"="UI: Post Action" ("State(s) in Front (\"\")"), "State(s) in (\"\")"=w292) -> ("States Out"=w293:string)  [unwired: 13 in]
        n110 = Not(x=w288) -> (.not. x?=w294:bool)
        n111 = Bundle By Name(cluster=w290, "Success"=w294) -> (w295:T3)
      }
    }
  }
  "Error out" <- w7
